vi "Config ARB Segment Trigger.vi"(0 "VISA Resource Name":refnum<visa-resource-name>, 5 "Type (1: Continuous)":enum16{"Single", "Continuous"}(ring)=enum."Continuous", 11 "error in (no error)":errorcluster {"code" format="%.0x"}) -> (4 "VISA Resource Name Out":refnum<visa-resource-name>, 15 "error out":errorcluster {"code" format="%.0x"})   [LabVIEW 2012, in "Agilent ESG Series.lvlib"]
doc: "This VI customizes the segment advance trigger type setting.\n\nNotes:\n(1) This VI is valid only on instrument E4438C with option 001/601 or 002/602."
uses:
  <instrlib>/Agilent ESG Series/Agilent ESG Series.lvlib
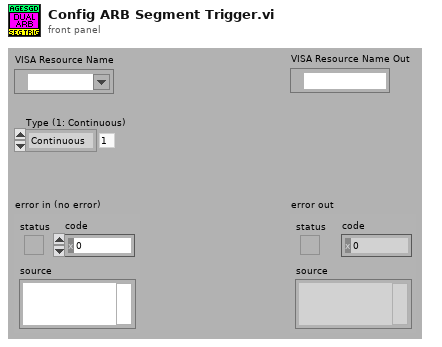
[diagram p1: front panel]
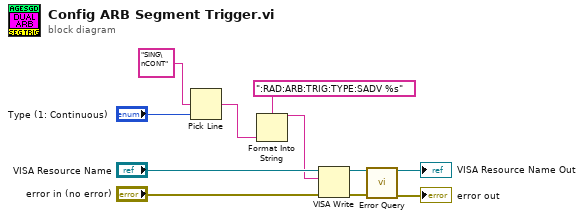
[diagram p0: block diagram]
diagram:
  n1 = Pick Line(multi-line string="SING\nCONT", line index="Type (1: Continuous)") -> (output string=w4:string)  [unwired: 1 in]
  n2 = Format Into String(format string=":RAD:ARB:TRIG:TYPE:SADV %s", w4) -> (resulting string=w3:string)  [unwired: 2 in, 1 out]
  n3 = VISA Write(VISA resource name="VISA Resource Name", write buffer=w3, error in (no error)="error in (no error)") -> (VISA resource name out=w7:refnum<visa-resource-name>, error out=w6:errorcluster)  [unwired: 1 out]
  n4 = call <instrlib>:"Error Query.vi"("VISA Resource Name"=w7, "error in (no error)"=w6) -> ("VISA Resource Name Out"=→"VISA Resource Name Out":refnum<visa-resource-name>, "error out"=→"error out":errorcluster)  [unwired: 10 in, 2 out]
